vi "PH_PPPA_PowerUnit.ProcCases.vi"(0 "i ref in":refnum<vi>, 1 "selector":string, 2 "Data":T1, 3 "call cluster":T2={"Object"="", "Selector"="", "CallType"=enum."synchronous", "Async Object"="", "Async Selector"="", "Data Descriptor"="", "Data"=[], "Error #"=0, "Expire"=0}, 5 "error in (no error)":errorcluster) -> (14 "i ref out":refnum<vi>, 17 "answer cluster":T2={"Object"="", "Selector"="", "CallType"=enum."synchronous", "Async Object"="", "Async Selector"="", "Data Descriptor"="", "Data"=[], "Error #"=0, "Expire"=0}, 19 "error out":errorcluster)   [LabVIEW 2014, in "PH_PPPA_PowerUnit.lvlib"]
doc: "This method is called by a process from within the default case in the event loop. The methods of a class that are linked to events will be called from THIS method. Add your code here."
uses:
  PH_PPPA_PowerUnit.lvlib
  CSCore/CSSystem/CoreDefs/CoreDefs.call_type.ctl
  CSCore/BaseProcess/BaseProcess.descriptor string definition.ctl
  CSCore/CSSystem/CoreDefs/CoreDefs.rawDataType.ctl
  PH_PowerUnit_BaseClass/PH_PowerUnit_BaseClass.SM States.ctl
  CSCore/CSSystem/CoreLib/CoreLib.string 2 byte array.vi
  CSCore/CSSystem/CoreLib/CoreLib.byte array 2 double.vi
  CSCore/CSSystem/CoreLib/CoreLib.byte array 2 short.vi
  CSCore/BaseProcess/BaseProcess.lvlib
  CSCore/CSSystem/CoreLib/CoreLib.lvlib
  CSCore/CAEObj/CAEObj.lvlib
  PH_Common/PH_Common.lvlib
  PH_StatusHandler/PH_StatusHandler.lvlib
  PH_PSDBWriter/PH_PSDBWriter.lvlib
  CSCore/BaseSM/BaseSM.lvlib
  PH_PowerUnit_BaseClass/PH_PowerUnit_BaseClass.lvlib
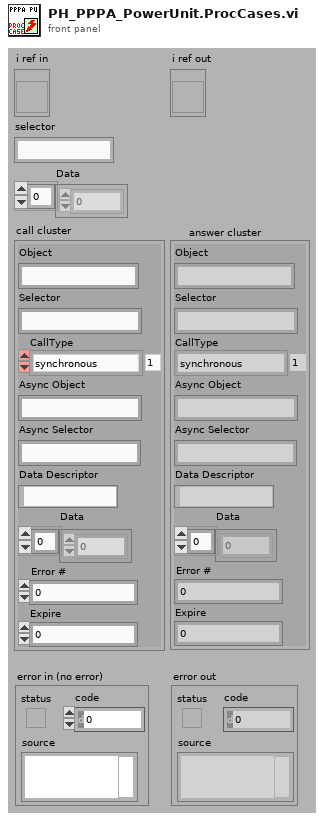
[diagram p1: front panel]
types:
  T1 = typedef "CoreDefs.rawDataType.ctl" = i8[]
  T2 = typedef "CoreDefs.call_type.ctl" = cluster{"Object":string, "Selector":string, "CallType":enum16{"simple", "synchronous", "asynchronous"}, "Async Object":string, "Async Selector":string, "Data Descriptor":T3, "Data":T1, "Error #":i32, "Expire":u32}
  T3 = typedef "BaseProcess.lvlib/BaseProcess.descriptor string definition.ctl" = string
  T4 = typedef "PH_PowerUnit_BaseClass.lvlib/PH_PowerUnit_BaseClass.SM States.ctl" = enum16{".", "Stand by", "Switch PU on", "Configure", "Set Default Voltage", "Set STANDBY", "Set READY", "Wait for Shot Cmd", "Open Dump Rods", "Open Ross Relais", "Close Ross Relais", "Switch PSU on", "Switch PSU off", "Charge", "Switch GD Channel on", "Close Dump Rods", "Rods-TO", "RR-TO", "PSU-TO", "Trigger-TO"}
  T5 = typedef "PH_PowerUnit_BaseClass.lvlib/PH_PowerUnit_BaseClass.i attribute.ctl" = cluster{"Constructor finished":bool, "PU":cluster{"In use":bool, "Service ID in use":i32, "GUI Ref":refnum<vi>}, "Enabling":cluster{"State":T6, "GUI Ref":refnum<vi>}, "Timing":cluster{"Last Shot":dbl, "Time between Shots [Sec]":dbl, "Waiting Time over?":bool, "Service ID Waiting Time":i32, "GUI Ref":refnum<vi>, "Instance":cluster{"Status":T7, "linked?":bool, "GUI Ref":refnum<vi>}}, "Sequencer":cluster{"SM State":string, "GUI Ref":refnum<vi>, "linked":bool}, "Subscribed Trendmssgs":cluster{"Tagname":string, "Status":T7, "linked?":bool, "Shot Condition":T7, "GUI Ref":refnum<vi>}[], "PP PU":T8, "Default Voltage (V)":dbl, "GUI Refs":T9, "PSDB data":cluster{"Shot Voltage [V]":dbl, "State TO SM":T4, "Write 2 early":bool}, "State TO SM":T4}
  T6 = typedef "PH_SystemInformation.lvlib/PH_SystemInformationEnabling State.ctl" = i32
  T7 = typedef "PH_StatusHandler.lvlib/PH_StatusHandler.Status.ctl" = i16
  T8 = typedef "PH_PP_Common.lvlib/PH_PP_Common.PUs.ctl" = enum16{"no Info", "PA-19mm-1", "PA-19mm-2", "PA-45mm-PILC", "PA-45mm-MAIN", "MA-PU-1", "MA-PU-2", "MA-PU-3", "MA-PU-4", "MA-PU-5", "MA-PU-6", "MA-FR", "MA-PILC", "PA-45mm-DP"}
  T9 = typedef "PH_PowerUnit_BaseClass.lvlib/PH_PowerUnit_BaseClass.GUI Refs.ctl" = cluster{"Delete Inst":refnum<vi>, "State TO SM":refnum<vi>, "State SM":refnum<vi>, "Fire":refnum<vi>}
  T10 = typedef "PH_PPPA_PowerUnit.lvlib/PH_PPPA_PowerUnit.i attribute.ctl" = cluster{"GUI Refs":cluster{"Ignitron":refnum<vi>, "Rossrelais":refnum<vi>, "Set Voltage":refnum<vi>, "PSU":refnum<vi>, "EOC":refnum<vi>, "Trigger":refnum<vi>}, "Ignitron":T11, "PSU":T12, "Dump Ross Relais":T13, "Trigger":cluster{"State Device":T7, "linked?":bool}, "Timing Settings":cluster{"Prdc Fast?":bool, "Default Value Periodic Interval":i32, "Mercury on since":dbl, "Warm up Time Mercury [s]":dbl}, "Set Voltage [V]":dbl, "19er Ignitionbox":string}
  T11 = typedef "PH_PP_Common.lvlib/PH_PP_Common.Ignitron Attributes.ctl" = cluster{"State Device":T7, "linked?":bool}
  T12 = typedef "PH_PP_Common.lvlib/PH_PP_Common.PSU Attributes.ctl" = cluster{"lower limit [V]":dbl, "upper limit [V]":dbl, "Voltage set":bool, "State Device":T7, "linked?":bool}
  T13 = typedef "PH_PP_Common.lvlib/PH_PP_Common.Ross Relais Attributes.ctl" = cluster{"State Device":T7, "linked?":bool}
  T14 = typedef "PH_PSDBWriter.lvlib/PH_PSDBWriter.PHELIX-Subsystems.ctl" = i32
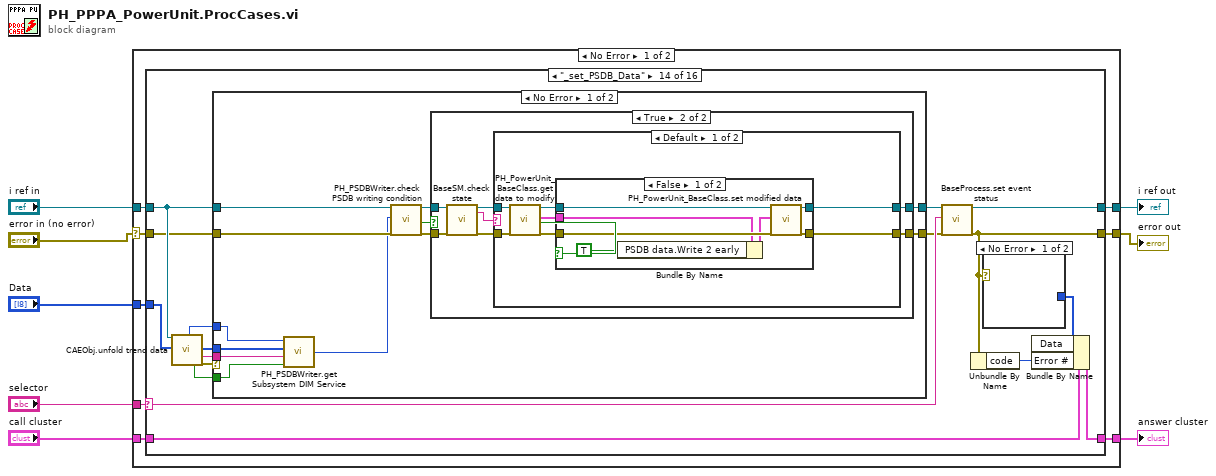
[diagram p0: block diagram]
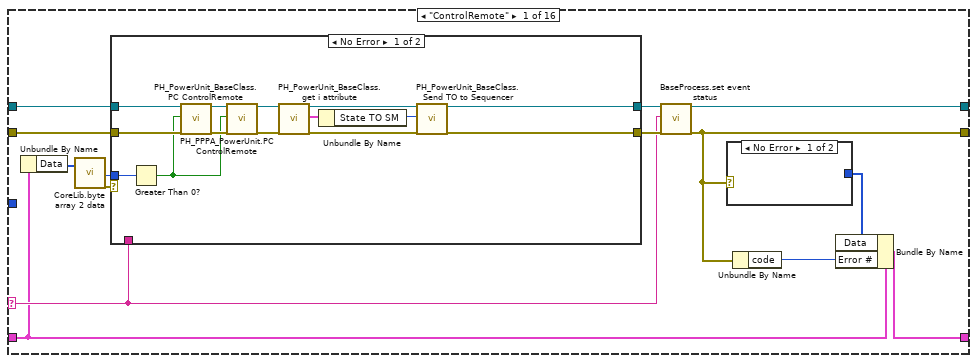
[diagram p2: hidden frame]
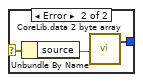
[diagram p3: hidden frame]
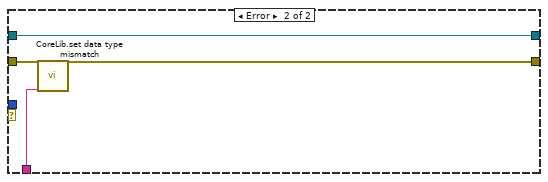
[diagram p4: hidden frame]
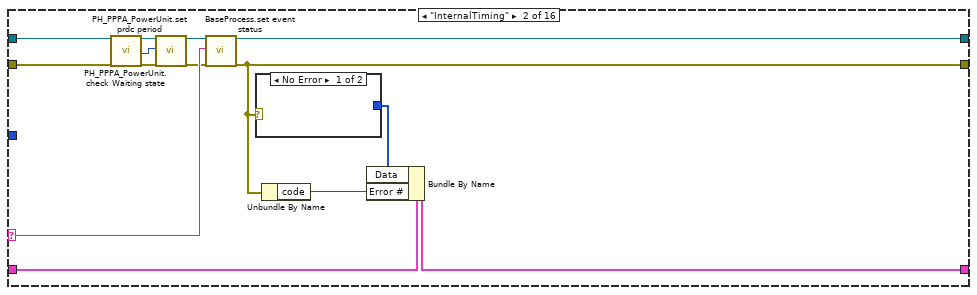
[diagram p5: hidden frame]
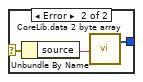
[diagram p6: hidden frame]
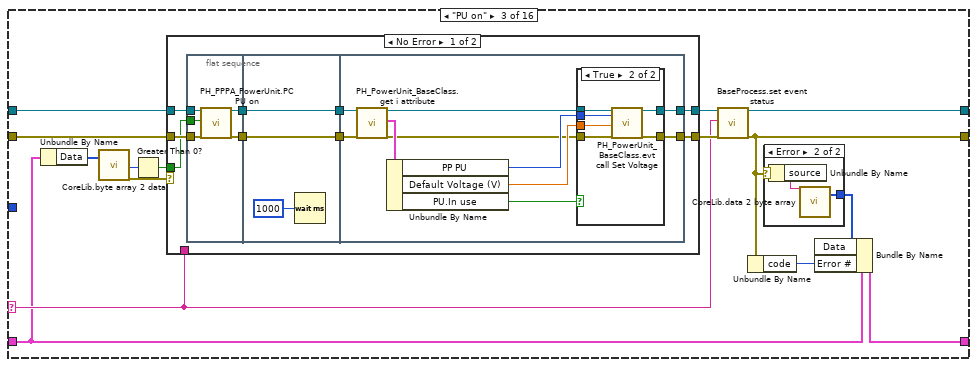
[diagram p7: hidden frame]
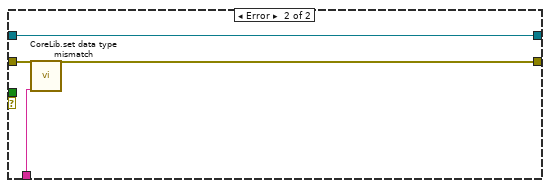
[diagram p10: hidden frame]
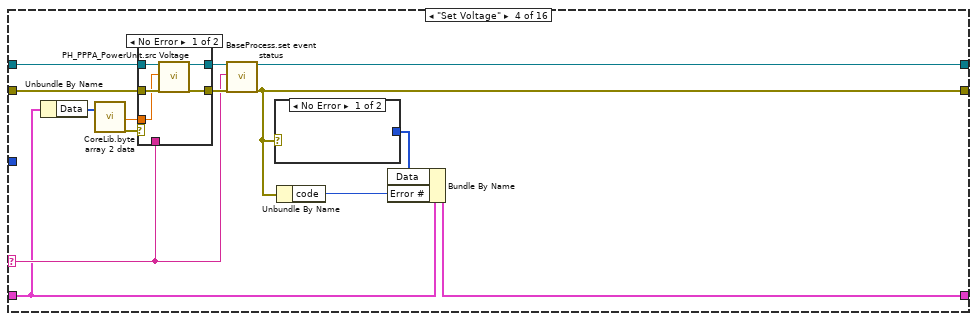
[diagram p11: hidden frame]
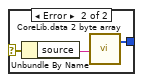
[diagram p12: hidden frame]
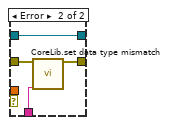
[diagram p13: hidden frame]
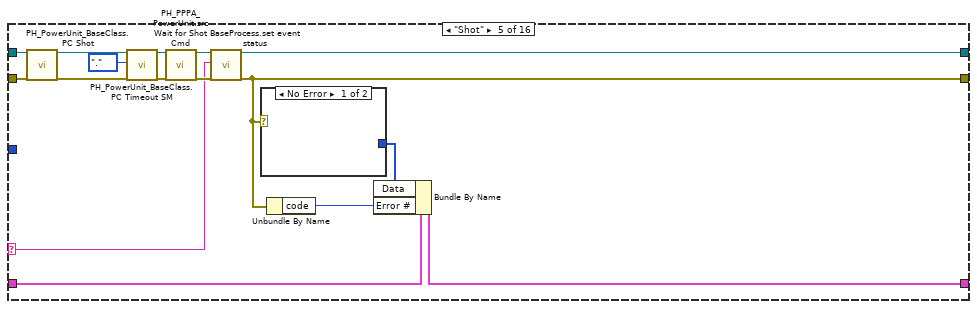
[diagram p14: hidden frame]
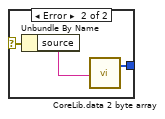
[diagram p15: hidden frame]
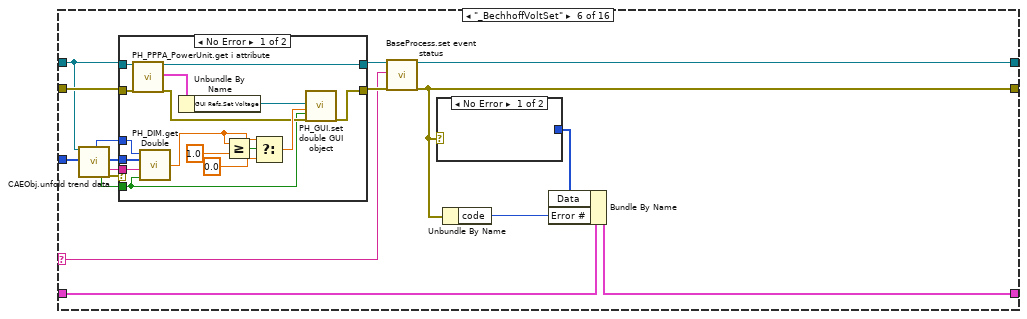
[diagram p16: hidden frame]
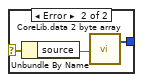
[diagram p17: hidden frame]
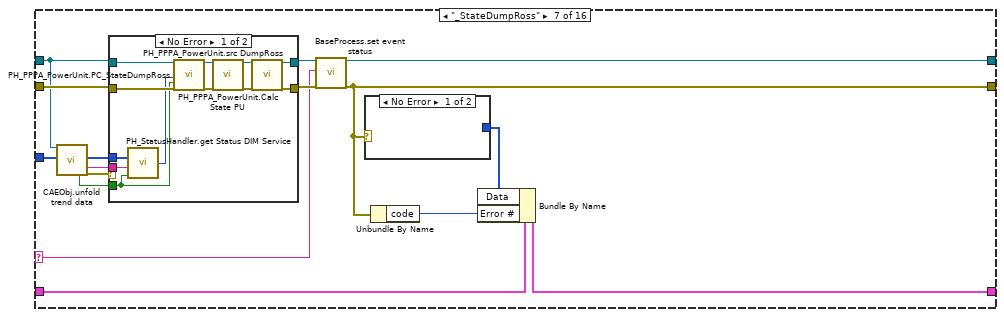
[diagram p19: hidden frame]
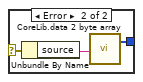
[diagram p20: hidden frame]
diagram:
  n1 = case shown="No Error" "error in (no error)" {
    selector: "error in (no error)" -> [w9 w589]
    tunnel: "selector" -> [w16 _]
    tunnel: [w15 w588] -> w7
    tunnel: "call cluster" -> [w14 w588]
    tunnel: "i ref in" -> [w13 w590]
    tunnel: [w12 w590] -> w4
    tunnel: [w11 w589] -> w3
    tunnel: "Data" -> [w10 _]
    frame No Error {
      n2 = case shown="\"_set_PSDB_Data\"" w16 {
        selector: w16 -> [w19 w60 w75 w133 w155 w180 w217 w250 w285 w338 w375 w404 w436 w489 w555 w580]
        tunnel: w13 -> [w30 w57 w83 w139 w167 w176 w213 w246 w279 w334 w369 w402 w435 w482 w548 w585]
        tunnel: [w21 w62 w77 w132 w157 w182 w220 w252 w287 w340 w374 w408 w440 w493 w559 w584] -> w12
        tunnel: w14 -> [w18 w59 w74 w130 w154 w179 w216 w249 w284 w337 w372 w406 w438 w491 w557 w578]
        tunnel: [w17 w58 w73 w129 w153 w178 w215 w248 w283 w336 w371 w405 w437 w490 w556 w581] -> w15
        tunnel: w9 -> [w29 w56 w82 w138 w166 w187 w224 w257 w278 w333 w380 w413 w445 w481 w547 w583]
        tunnel: [w20 w61 w76 w131 w156 w181 w219 w251 w286 w339 w373 w407 w439 w492 w558 w582] -> w11
        tunnel: w10 -> [_ _ _ _ _ w177 w214 w247 w282 w335 w370 w403 w434 w483 w549 w579]
        frame "ControlRemote" {
          n3 = Unbundle By Name(w18) -> ("Data"=w28:T1)
          n4 = call-poly "CoreLib.byte array 2 data.vi"("byteArray"=w28) -> ("i16"=w26:i16, "error out"=w27:errorcluster)  [unwired: 16 in, 1 out]
          n5 = case shown="No Error" w27 {
            tunnel: [w42 w51] -> w22
            tunnel: w30 -> [w47 w51]
            tunnel: w29 -> [w46 w50]
            tunnel: [w41 w49] -> w23
            tunnel: w19 -> [_ w48]
            tunnel: w26 -> [w35 _]
            frame No Error {
              n6 = Greater Than 0?(x=w35) -> (x > 0?=w34:bool)
              n7 = call "PH_PPPA_PowerUnit.PC ControlRemote.vi"("i ref in"=w47, "Remote Controlled?"=w34, "error in (no error)"=w46) -> ("i ref out"=w39:refnum<vi>, "error out"=w37:errorcluster)  [unwired: 15 in]
              n8 = call "PH_PowerUnit_BaseClass.PC ControlRemote.vi"("i ref in"=w39, "Remote controlled?"=w34, "error in (no error)"=w37) -> ("i ref out"=w38:refnum<vi>, "error out"=w36:errorcluster)  [unwired: 15 in]
              n9 = call "PH_PowerUnit_BaseClass.get i attribute.vi"("i ref in"=w38, "error in (no error)"=w36) -> ("i ref out"=w44:refnum<vi>, "i attribute"=w45:T5, "error out"=w40:errorcluster)  [unwired: 15 in]
              n10 = Unbundle By Name(w45) -> ("State TO SM"=w43:T4)
              n11 = call "PH_PowerUnit_BaseClass.Send TO to Sequencer.vi"("VI in"=w44, "State TO SM"=w43, "error in (no error)"=w40) -> ("VI out"=w42:refnum<vi>, "error out"=w41:errorcluster)  [unwired: 15 in]
            }
            frame Error {
              n12 = call "CoreLib.set data type mismatch.vi"("error in (no error)"=w50, "error source"=w48) -> ("error out"=w49:errorcluster)  [unwired: 17 in]
            }
          }
          n13 = call "BaseProcess.set event status.vi"("i ref in"=w22, "EventStatus"=w19, "error in (no error)"=w23) -> ("i ref out"=w21:refnum<vi>, "error out"=w20:errorcluster)  [unwired: 14 in, 1 out]
          n14 = case shown="No Error" w20 {
            selector: w20 -> [_ w33]
            tunnel: [_ w31] -> w24
            frame No Error {
            }
            frame Error {
              n15 = Unbundle By Name(w33) -> ("source"=w32:string)
              n16 = call-poly "CoreLib.data 2 byte array.vi"("string"=w32) -> ("byteArray out"=w31:T1)  [unwired: 18 in]
            }
          }
          n17 = Unbundle By Name(w20) -> ("code"=w25:i32)
          n18 = Bundle By Name(cluster=w18, "Data"=w24, "Error #"=w25) -> (w17:T2)
        }
        frame "InternalTiming" {
          n19 = call "PH_PPPA_PowerUnit.check Waiting state.vi"("i ref in"=w57, "error in (no error)"=w56) -> ("i ref out"=w55:refnum<vi>, "Waiting Time (s)"=w65:i32, "error out"=w54:errorcluster)  [unwired: 15 in]
          n20 = call "PH_PPPA_PowerUnit.set  prdc period.vi"("i ref in"=w55, "Waiting Time (s)"=w65, "error in (no error)"=w54) -> ("i ref out"=w53:refnum<vi>, "error out"=w52:errorcluster)  [unwired: 15 in]
          n21 = call "BaseProcess.set event status.vi"("i ref in"=w53, "EventStatus"=w60, "error in (no error)"=w52) -> ("i ref out"=w62:refnum<vi>, "error out"=w61:errorcluster)  [unwired: 14 in, 1 out]
          n22 = case shown="No Error" w61 {
            selector: w61 -> [_ w68]
            tunnel: [_ w66] -> w63
            frame No Error {
            }
            frame Error {
              n23 = Unbundle By Name(w68) -> ("source"=w67:string)
              n24 = call-poly "CoreLib.data 2 byte array.vi"("string"=w67) -> ("byteArray out"=w66:T1)  [unwired: 18 in]
            }
          }
          n25 = Unbundle By Name(w61) -> ("code"=w64:i32)
          n26 = Bundle By Name(cluster=w59, "Data"=w63, "Error #"=w64) -> (w58:T2)
        }
        frame "PU on" {
          n27 = Unbundle By Name(w74) -> ("Data"=w72:T1)
          n28 = call-poly "CoreLib.byte array 2 data.vi"("byteArray"=w72) -> ("i16"=w71:i16, "error out"=w69:errorcluster)  [unwired: 16 in, 1 out]
          n29 = Greater Than 0?(x=w71) -> (x > 0?=w70:bool)
          n30 = case shown="No Error" w69 {
            tunnel: w83 -> [w95 w123]
            tunnel: [w93 w123] -> w78
            tunnel: w82 -> [w94 w125]
            tunnel: [w92 w124] -> w79
            tunnel: w75 -> [_ w122]
            tunnel: w70 -> [w91 _]
            frame No Error {
              n31 = flat-sequence {
                tunnel: w95 -> [w100]
                tunnel: w94 -> [w99]
                tunnel: w91 -> [w96]
                tunnel: [w98] -> w90
                tunnel: [w97] -> w89
                tunnel: w90 -> [w103]
                tunnel: w89 -> [w102]
                tunnel: [w103] -> w88
                tunnel: [w102] -> w87
                tunnel: [w110] -> w92
                tunnel: [w111] -> w93
                tunnel: w88 -> [w113]
                tunnel: w87 -> [w112]
                frame #0 {
                  n32 = call "PH_PPPA_PowerUnit.PC PU on.vi"("i ref in"=w100, "PU on"=w96, "error in (no error)"=w99) -> ("i ref out"=w98:refnum<vi>, "error out"=w97:errorcluster)  [unwired: 15 in]
                }
                frame #1 {
                  n33 = Wait (ms)(milliseconds to wait=u32 1000) -> ()  [unwired: 1 out]
                }
                frame #2 {
                  n34 = call "PH_PowerUnit_BaseClass.get i attribute.vi"("i ref in"=w113, "error in (no error)"=w112) -> ("i ref out"=w105:refnum<vi>, "i attribute"=w109:T5, "error out"=w104:errorcluster)  [unwired: 15 in]
                  n35 = Unbundle By Name(w109) -> ("PP PU"=w106:T8, "Default Voltage (V)"=w107:dbl, "PU.In use"=w108:bool)
                  n36 = case shown="True" w108 {
                    tunnel: w105 -> [w115 w121]
                    tunnel: [w115 w120] -> w111
                    tunnel: w104 -> [w114 w119]
                    tunnel: [w114 w118] -> w110
                    tunnel: w107 -> [_ w117]
                    tunnel: w106 -> [_ w116]
                    frame False {
                    }
                    frame True {
                      n37 = call "PH_PowerUnit_BaseClass.evt call Set Voltage.vi"("i ref in"=w121, "PowerUnit"=w116, "Voltage [V]"=w117, "error in (no error)"=w119) -> ("i ref out"=w120:refnum<vi>, "error out"=w118:errorcluster)  [unwired: 14 in]
                    }
                  }
                }
              }
            }
            frame Error {
              n38 = call "CoreLib.set data type mismatch.vi"("error in (no error)"=w125, "error source"=w122) -> ("error out"=w124:errorcluster)  [unwired: 17 in]
            }
          }
          n39 = call "BaseProcess.set event status.vi"("i ref in"=w78, "EventStatus"=w75, "error in (no error)"=w79) -> ("i ref out"=w77:refnum<vi>, "error out"=w76:errorcluster)  [unwired: 14 in, 1 out]
          n40 = Unbundle By Name(w76) -> ("code"=w81:i32)
          n41 = case shown="Error" w76 {
            selector: w76 -> [_ w86]
            tunnel: [_ w84] -> w80
            frame No Error {
            }
            frame Error {
              n42 = Unbundle By Name(w86) -> ("source"=w85:string)
              n43 = call-poly "CoreLib.data 2 byte array.vi"("string"=w85) -> ("byteArray out"=w84:T1)  [unwired: 18 in]
            }
          }
          n44 = Bundle By Name(cluster=w74, "Data"=w80, "Error #"=w81) -> (w73:T2)
        }
        frame "Set Voltage" {
          n45 = Unbundle By Name(w130) -> ("Data"=w128:T1)
          n46 = call-poly "CoreLib.byte array 2 data.vi"("byteArray"=w128) -> ("d64"=w127:dbl, "error out"=w126:errorcluster)  [unwired: 16 in, 1 out]
          n47 = case shown="No Error" w126 {
            tunnel: w139 -> [w147 w149]
            tunnel: [w145 w149] -> w134
            tunnel: w138 -> [w146 w151]
            tunnel: [w144 w150] -> w135
            tunnel: w133 -> [_ w148]
            tunnel: w127 -> [w143 _]
            frame No Error {
              n48 = call "PH_PPPA_PowerUnit.src Voltage.vi"("i ref in"=w147, "Voltage [V]"=w143, "error in (no error)"=w146) -> ("i ref out"=w145:refnum<vi>, "error out"=w144:errorcluster)  [unwired: 15 in]
            }
            frame Error {
              n49 = call "CoreLib.set data type mismatch.vi"("error in (no error)"=w151, "error source"=w148) -> ("error out"=w150:errorcluster)  [unwired: 17 in]
            }
          }
          n50 = call "BaseProcess.set event status.vi"("i ref in"=w134, "EventStatus"=w133, "error in (no error)"=w135) -> ("i ref out"=w132:refnum<vi>, "error out"=w131:errorcluster)  [unwired: 14 in, 1 out]
          n51 = case shown="No Error" w131 {
            selector: w131 -> [_ w142]
            tunnel: [_ w140] -> w136
            frame No Error {
            }
            frame Error {
              n52 = Unbundle By Name(w142) -> ("source"=w141:string)
              n53 = call-poly "CoreLib.data 2 byte array.vi"("string"=w141) -> ("byteArray out"=w140:T1)  [unwired: 18 in]
            }
          }
          n54 = Unbundle By Name(w131) -> ("code"=w137:i32)
          n55 = Bundle By Name(cluster=w130, "Data"=w136, "Error #"=w137) -> (w129:T2)
        }
        frame "Shot" {
          n56 = call "PH_PowerUnit_BaseClass.PC Shot.vi"("i ref in"=w167, "error in (no error)"=w166) -> ("i ref out"=w165:refnum<vi>, "error out"=w164:errorcluster)  [unwired: 16 in]
          n57 = call "PH_PowerUnit_BaseClass.PC Timeout SM.vi"("VI in"=w165, "Timeout SM"=PH_PowerUnit_BaseClass.SM_States.".", "error in (no error)"=w164) -> ("VI out"=w162:refnum<vi>, "error out"=w163:errorcluster)  [unwired: 15 in]
          n58 = call "PH_PPPA_PowerUnit.src Wait for Shot Cmd.vi"("i ref in"=w162, "error in (no error)"=w163) -> ("i ref out"=w158:refnum<vi>, "error out"=w159:errorcluster)  [unwired: 16 in]
          n59 = call "BaseProcess.set event status.vi"("i ref in"=w158, "EventStatus"=w155, "error in (no error)"=w159) -> ("i ref out"=w157:refnum<vi>, "error out"=w156:errorcluster)  [unwired: 14 in, 1 out]
          n60 = case shown="No Error" w156 {
            selector: w156 -> [_ w170]
            tunnel: [_ w168] -> w160
            frame No Error {
            }
            frame Error {
              n61 = Unbundle By Name(w170) -> ("source"=w169:string)
              n62 = call-poly "CoreLib.data 2 byte array.vi"("string"=w169) -> ("byteArray out"=w168:T1)  [unwired: 18 in]
            }
          }
          n63 = Unbundle By Name(w156) -> ("code"=w161:i32)
          n64 = Bundle By Name(cluster=w154, "Data"=w160, "Error #"=w161) -> (w153:T2)
        }
        frame "_BechhoffVoltSet" {
          n65 = call "CAEObj.unfold trend data.vi"("i ref in"=w176, "raw trend data"=w177) -> ("quality"=w171:i32, "no link"=w172:bool, "data"=w173:i8[], "typeDescriptor"=w174:string, "error out"=w175:errorcluster)  [unwired: 9 in, 4 out]
          n66 = case shown="No Error" w175 {
            tunnel: w176 -> [w206 w208]
            tunnel: [w201 w208] -> w183
            tunnel: w187 -> [w205 w207]
            tunnel: [w192 w207] -> w184
            tunnel: w174 -> [w198 _]
            tunnel: w173 -> [w197 _]
            tunnel: w172 -> [w191 _]
            tunnel: w171 -> [w196 _]
            frame No Error {
              n67 = call "PH_PPPA_PowerUnit.get i attribute.vi"("i ref in"=w206, "error in (no error)"=w205) -> ("i ref out"=w201:refnum<vi>, "i attribute"=w204:T10, "error out"=w193:errorcluster)  [unwired: 15 in]
              n68 = call "PH_DIM.get Double.vi"("no link"=w191, "typeDescriptor"=w198, "data"=w197, "quality"=w196) -> ("Value"=w200:dbl)
              n69 = Unbundle By Name(w204) -> ("GUI Refs.Set Voltage"=w194:refnum<vi>)
              n70 = Greater Or Equal?(x=w200, y=1.0) -> (x >= y?=w199:bool)
              n71 = Select(t=w200, s=w199, f=0.0) -> (s? t:f=w195:dbl)
              n72 = call "PH_GUI.set double GUI object.vi"("GUI object Ref"=w194, "value"=w195, "blinking (false)"=w191, "error in (no error)"=w193) -> ("error out"=w192:errorcluster)  [unwired: 15 in]
            }
            frame Error {
            }
          }
          n73 = call "BaseProcess.set event status.vi"("i ref in"=w183, "EventStatus"=w180, "error in (no error)"=w184) -> ("i ref out"=w182:refnum<vi>, "error out"=w181:errorcluster)  [unwired: 14 in, 1 out]
          n74 = case shown="No Error" w181 {
            selector: w181 -> [_ w190]
            tunnel: [_ w188] -> w185
            frame No Error {
            }
            frame Error {
              n75 = Unbundle By Name(w190) -> ("source"=w189:string)
              n76 = call-poly "CoreLib.data 2 byte array.vi"("string"=w189) -> ("byteArray out"=w188:T1)  [unwired: 18 in]
            }
          }
          n77 = Unbundle By Name(w181) -> ("code"=w186:i32)
          n78 = Bundle By Name(cluster=w179, "Data"=w185, "Error #"=w186) -> (w178:T2)
        }
        frame "_StateDumpRoss" {
          n79 = call "CAEObj.unfold trend data.vi"("i ref in"=w213, "raw trend data"=w214) -> ("no link"=w209:bool, "data"=w211:i8[], "typeDescriptor"=w212:string, "error out"=w210:errorcluster)  [unwired: 9 in, 5 out]
          n80 = case shown="No Error" w210 {
            tunnel: w213 -> [w239 w241]
            tunnel: [w233 w241] -> w218
            tunnel: w224 -> [w238 w240]
            tunnel: [w234 w240] -> w221
            tunnel: w212 -> [w237 _]
            tunnel: w211 -> [w236 _]
            tunnel: w209 -> [w228 _]
            frame No Error {
              n81 = call "PH_StatusHandler.get Status DIM Service.vi"("no link"=w228, "typeDescriptor"=w237, "data"=w236) -> ("Status"=w235:T7)  [unwired: 1 in]
              n82 = call "PH_PPPA_PowerUnit.PC_StateDumpRoss.vi"("i ref in"=w239, "Dump Ross State"=w235, "not linked"=w228, "error in (no error)"=w238) -> ("i ref out"=w232:refnum<vi>, "error out"=w230:errorcluster)  [unwired: 14 in]
              n83 = call "PH_PPPA_PowerUnit.Calc State PU.vi"("i ref in"=w232, "error in (no error)"=w230) -> ("i ref out"=w231:refnum<vi>, "error out"=w229:errorcluster)  [unwired: 16 in]
              n84 = call "PH_PPPA_PowerUnit.src DumpRoss.vi"("i ref in"=w231, "error in (no error)"=w229) -> ("i ref out"=w233:refnum<vi>, "error out"=w234:errorcluster)  [unwired: 16 in]
            }
            frame Error {
            }
          }
          n85 = call "BaseProcess.set event status.vi"("i ref in"=w218, "EventStatus"=w217, "error in (no error)"=w221) -> ("i ref out"=w220:refnum<vi>, "error out"=w219:errorcluster)  [unwired: 14 in, 1 out]
          n86 = case shown="No Error" w219 {
            selector: w219 -> [_ w227]
            tunnel: [_ w225] -> w222
            frame No Error {
            }
            frame Error {
              n87 = Unbundle By Name(w227) -> ("source"=w226:string)
              n88 = call-poly "CoreLib.data 2 byte array.vi"("string"=w226) -> ("byteArray out"=w225:T1)  [unwired: 18 in]
            }
          }
          n89 = Unbundle By Name(w219) -> ("code"=w223:i32)
          n90 = Bundle By Name(cluster=w216, "Data"=w222, "Error #"=w223) -> (w215:T2)
        }
        frame "_StateIgni" {
          n91 = call "CAEObj.unfold trend data.vi"("i ref in"=w246, "raw trend data"=w247) -> ("no link"=w242:bool, "data"=w244:i8[], "typeDescriptor"=w243:string, "error out"=w245:errorcluster)  [unwired: 9 in, 5 out]
          n92 = case shown="No Error" w245 {
            tunnel: w246 -> [w268 w272]
            tunnel: [w270 w272] -> w253
            tunnel: w257 -> [w266 w271]
            tunnel: [w269 w271] -> w254
            tunnel: w244 -> [w264 _]
            tunnel: w243 -> [w263 _]
            tunnel: w242 -> [w261 _]
            frame No Error {
              n93 = call "PH_StatusHandler.get Status DIM Service.vi"("no link"=w261, "typeDescriptor"=w263, "data"=w264) -> ("Status"=w262:T7)  [unwired: 1 in]
              n94 = call "PH_PPPA_PowerUnit.PC_StateIgni.vi"("i ref in"=w268, "Igni Status"=w262, "not linked?"=w261, "error in (no error)"=w266) -> ("i ref out"=w267:refnum<vi>, "error out"=w265:errorcluster)  [unwired: 14 in]
              n95 = call "PH_PPPA_PowerUnit.Calc State PU.vi"("i ref in"=w267, "error in (no error)"=w265) -> ("i ref out"=w270:refnum<vi>, "error out"=w269:errorcluster)  [unwired: 16 in]
            }
            frame Error {
            }
          }
          n96 = call "BaseProcess.set event status.vi"("i ref in"=w253, "EventStatus"=w250, "error in (no error)"=w254) -> ("i ref out"=w252:refnum<vi>, "error out"=w251:errorcluster)  [unwired: 14 in, 1 out]
          n97 = case shown="No Error" w251 {
            selector: w251 -> [_ w260]
            tunnel: [_ w258] -> w255
            frame No Error {
            }
            frame Error {
              n98 = Unbundle By Name(w260) -> ("source"=w259:string)
              n99 = call-poly "CoreLib.data 2 byte array.vi"("string"=w259) -> ("byteArray out"=w258:T1)  [unwired: 18 in]
            }
          }
          n100 = Unbundle By Name(w251) -> ("code"=w256:i32)
          n101 = Bundle By Name(cluster=w249, "Data"=w255, "Error #"=w256) -> (w248:T2)
        }
        frame "_MercuryOnSince" {
          n102 = call "CAEObj.unfold trend data.vi"("i ref in"=w279, "raw trend data"=w282) -> ("quality"=w277:i32, "no link"=w276:bool, "data"=w273:i8[], "typeDescriptor"=w274:string, "error out"=w275:errorcluster)  [unwired: 9 in, 4 out]
          n103 = case shown="No Error" w275 {
            tunnel: w279 -> [w302 w322]
            tunnel: [w297 w322] -> w280
            tunnel: w278 -> [w301 w321]
            tunnel: [w295 w321] -> w281
            tunnel: w273 -> [w300 _]
            tunnel: w274 -> [w299 _]
            tunnel: w276 -> [w290 _]
            tunnel: w277 -> [w294 _]
            frame No Error {
              n104 = call "PH_PPPA_PowerUnit.get data to modify.vi"("i ref in"=w302, "error in (no error)"=w301) -> ("i ref out"=w298:refnum<vi>, "i attribute"=w291:T10, "timed out"=w292:bool, "error out"=w296:errorcluster)  [unwired: 14 in]
              n105 = call "PH_DIM.get String.vi"("no link"=w290, "typeDescriptor"=w299, "data"=w300, "quality"=w294) -> ("Output String"=w293:string)
              n106 = case shown="False" w292 {
                tunnel: w298 -> [w311 w320]
                tunnel: [w310 w320] -> w297
                tunnel: w296 -> [w309 w319]
                tunnel: [w308 w319] -> w295
                tunnel: w293 -> [w307 _]
                tunnel: w291 -> [w306 _]
                tunnel: w290 -> [w304 _]
                frame False {
                  n107 = case shown="False" w304 {
                    tunnel: w307 -> [w314 _]
                    tunnel: [w313 9999.0] -> w303
                    frame False {
                      n108 = Match Pattern(string=w314, regular expression=" ") -> (before substring=w316:string, after substring=w315:string)  [unwired: 1 in, 2 out]
                      n109 = call "PH_Strings.convert Time 1.vi"("Date"=w316, "Time"=w315) -> ("Time"=w312:timestamp)
                      n110 = To Double Precision Float(number=w312) -> (double precision float=w313:dbl)
                    }
                    frame True {
                    }
                  }
                  n111 = Bundle By Name(cluster=w306, "Timing Settings.Mercury on since"=w303) -> (w305:T10)
                  n112 = call "PH_PPPA_PowerUnit.set modified data.vi"("i ref in"=w311, "i attribute"=w305, "error in (no error)"=w309) -> ("i ref out"=w310:refnum<vi>, "error out"=w308:errorcluster)  [unwired: 15 in]
                }
                frame True {
                }
              }
            }
            frame Error {
            }
          }
          n113 = call "BaseProcess.set event status.vi"("i ref in"=w280, "EventStatus"=w285, "error in (no error)"=w281) -> ("i ref out"=w287:refnum<vi>, "error out"=w286:errorcluster)  [unwired: 14 in, 1 out]
          n114 = case shown="No Error" w286 {
            selector: w286 -> [_ w325]
            tunnel: [_ w323] -> w288
            frame No Error {
            }
            frame Error {
              n115 = Unbundle By Name(w325) -> ("source"=w324:string)
              n116 = call-poly "CoreLib.data 2 byte array.vi"("string"=w324) -> ("byteArray out"=w323:T1)  [unwired: 18 in]
            }
          }
          n117 = Unbundle By Name(w286) -> ("code"=w289:i32)
          n118 = Bundle By Name(cluster=w284, "Data"=w288, "Error #"=w289) -> (w283:T2)
        }
        frame "_LastShot" {
          n119 = call "CAEObj.unfold trend data.vi"("i ref in"=w334, "raw trend data"=w335) -> ("quality"=w329:i32, "no link"=w330:bool, "data"=w328:i8[], "typeDescriptor"=w326:string, "error out"=w327:errorcluster)  [unwired: 9 in, 4 out]
          n120 = case shown="No Error" w327 {
            tunnel: w334 -> [w344 w361]
            tunnel: [w350 w361] -> w332
            tunnel: w333 -> [w343 w360]
            tunnel: [w349 w360] -> w331
            tunnel: w328 -> [w352 _]
            tunnel: w326 -> [w351 _]
            tunnel: w330 -> [w346 _]
            tunnel: w329 -> [w348 _]
            frame No Error {
              n121 = call "PH_DIM.get String.vi"("no link"=w346, "typeDescriptor"=w351, "data"=w352, "quality"=w348) -> ("Output String"=w347:string)
              n122 = case shown="False" w346 {
                tunnel: w347 -> [w355 _]
                tunnel: [w353 9999.0] -> w345
                frame False {
                  n123 = Match Pattern(string=w355, regular expression=" ") -> (before substring=w357:string, after substring=w356:string)  [unwired: 1 in, 2 out]
                  n124 = call "PH_Strings.convert Time 1.vi"("Date"=w357, "Time"=w356) -> ("Time"=w354:timestamp)
                  n125 = To Double Precision Float(number=w354) -> (double precision float=w353:dbl)
                }
                frame True {
                }
              }
              n126 = call "PH_PowerUnit_BaseClass.set Last Shot.vi"("VI in"=w344, "Last Shot"=w345, "error in (no error)"=w343) -> ("VI out"=w350:refnum<vi>, "error out"=w349:errorcluster)  [unwired: 15 in]
            }
            frame Error {
            }
          }
          n127 = call "BaseProcess.set event status.vi"("i ref in"=w332, "EventStatus"=w338, "error in (no error)"=w331) -> ("i ref out"=w340:refnum<vi>, "error out"=w339:errorcluster)  [unwired: 14 in, 1 out]
          n128 = case shown="No Error" w339 {
            selector: w339 -> [_ w364]
            tunnel: [_ w362] -> w341
            frame No Error {
            }
            frame Error {
              n129 = Unbundle By Name(w364) -> ("source"=w363:string)
              n130 = call-poly "CoreLib.data 2 byte array.vi"("string"=w363) -> ("byteArray out"=w362:T1)  [unwired: 18 in]
            }
          }
          n131 = Unbundle By Name(w339) -> ("code"=w342:i32)
          n132 = Bundle By Name(cluster=w337, "Data"=w341, "Error #"=w342) -> (w336:T2)
        }
        frame "_StatePSU" {
          n133 = call "CAEObj.unfold trend data.vi"("i ref in"=w369, "raw trend data"=w370) -> ("no link"=w365:bool, "data"=w366:i8[], "typeDescriptor"=w367:string, "error out"=w368:errorcluster)  [unwired: 9 in, 5 out]
          n134 = case shown="No Error" w368 {
            tunnel: w369 -> [w395 w397]
            tunnel: [w388 w397] -> w376
            tunnel: w380 -> [w394 w396]
            tunnel: [w389 w396] -> w377
            tunnel: w367 -> [w393 _]
            tunnel: w366 -> [w392 _]
            tunnel: w365 -> [w390 _]
            frame No Error {
              n135 = call "PH_StatusHandler.get Status DIM Service.vi"("no link"=w390, "typeDescriptor"=w393, "data"=w392) -> ("Status"=w391:T7)  [unwired: 1 in]
              n136 = call "PH_PPPA_PowerUnit.PC_StatePSU.vi"("i ref in"=w395, "State PSU"=w391, "not linked?"=w390, "error in (no error)"=w394) -> ("i ref out"=w387:refnum<vi>, "error out"=w385:errorcluster)  [unwired: 14 in]
              n137 = call "PH_PPPA_PowerUnit.Calc State PU.vi"("i ref in"=w387, "error in (no error)"=w385) -> ("i ref out"=w386:refnum<vi>, "error out"=w384:errorcluster)  [unwired: 16 in]
              n138 = call "PH_PPPA_PowerUnit.src PSU.vi"("i ref in"=w386, "error in (no error)"=w384) -> ("i ref out"=w388:refnum<vi>, "error out"=w389:errorcluster)  [unwired: 16 in]
            }
            frame Error {
            }
          }
          n139 = call "BaseProcess.set event status.vi"("i ref in"=w376, "EventStatus"=w375, "error in (no error)"=w377) -> ("i ref out"=w374:refnum<vi>, "error out"=w373:errorcluster)  [unwired: 14 in, 1 out]
          n140 = case shown="No Error" w373 {
            selector: w373 -> [_ w383]
            tunnel: [_ w381] -> w378
            frame No Error {
            }
            frame Error {
              n141 = Unbundle By Name(w383) -> ("source"=w382:string)
              n142 = call-poly "CoreLib.data 2 byte array.vi"("string"=w382) -> ("byteArray out"=w381:T1)  [unwired: 18 in]
            }
          }
          n143 = Unbundle By Name(w373) -> ("code"=w379:i32)
          n144 = Bundle By Name(cluster=w372, "Data"=w378, "Error #"=w379) -> (w371:T2)
        }
        frame "_StateTrigger" {
          n145 = call "CAEObj.unfold trend data.vi"("i ref in"=w402, "raw trend data"=w403) -> ("no link"=w398:bool, "data"=w400:i8[], "typeDescriptor"=w399:string, "error out"=w401:errorcluster)  [unwired: 9 in, 5 out]
          n146 = case shown="No Error" w401 {
            tunnel: w402 -> [w428 w430]
            tunnel: [w421 w430] -> w409
            tunnel: w413 -> [w427 w429]
            tunnel: [w422 w429] -> w410
            tunnel: w400 -> [w426 _]
            tunnel: w399 -> [w425 _]
            tunnel: w398 -> [w423 _]
            frame No Error {
              n147 = call "PH_StatusHandler.get Status DIM Service.vi"("no link"=w423, "typeDescriptor"=w425, "data"=w426) -> ("Status"=w424:T7)  [unwired: 1 in]
              n148 = call "PH_PPPA_PowerUnit.PC_StateTrigger.vi"("i ref in"=w428, "Trigger Status"=w424, "not linked?"=w423, "error in (no error)"=w427) -> ("i ref out"=w420:refnum<vi>, "error out"=w418:errorcluster)  [unwired: 14 in]
              n149 = call "PH_PPPA_PowerUnit.Calc State PU.vi"("i ref in"=w420, "error in (no error)"=w418) -> ("i ref out"=w419:refnum<vi>, "error out"=w417:errorcluster)  [unwired: 16 in]
              n150 = call "PH_PPPA_PowerUnit.src Switch GD Channel on.vi"("i ref in"=w419, "error in (no error)"=w417) -> ("i ref out"=w421:refnum<vi>, "error out"=w422:errorcluster)  [unwired: 16 in]
            }
            frame Error {
            }
          }
          n151 = call "BaseProcess.set event status.vi"("i ref in"=w409, "EventStatus"=w404, "error in (no error)"=w410) -> ("i ref out"=w408:refnum<vi>, "error out"=w407:errorcluster)  [unwired: 14 in, 1 out]
          n152 = case shown="No Error" w407 {
            selector: w407 -> [_ w416]
            tunnel: [_ w414] -> w411
            frame No Error {
            }
            frame Error {
              n153 = Unbundle By Name(w416) -> ("source"=w415:string)
              n154 = call-poly "CoreLib.data 2 byte array.vi"("string"=w415) -> ("byteArray out"=w414:T1)  [unwired: 18 in]
            }
          }
          n155 = Unbundle By Name(w407) -> ("code"=w412:i32)
          n156 = Bundle By Name(cluster=w406, "Data"=w411, "Error #"=w412) -> (w405:T2)
        }
        frame "_setLimits" {
          n157 = call "CAEObj.unfold trend data.vi"("i ref in"=w435, "raw trend data"=w434) -> ("no link"=w431:bool, "data"=w433:i8[], "error out"=w432:errorcluster)  [unwired: 9 in, 6 out]
          n158 = case shown="No Error" w432 {
            tunnel: w435 -> [w450 w478]
            tunnel: [w456 w478] -> w441
            tunnel: w445 -> [w449 w477]
            tunnel: [w455 w477] -> w442
            tunnel: w433 -> [w452 _]
            tunnel: w431 -> [w451 _]
            frame No Error {
              n159 = case shown="False" w451 {
                tunnel: [w465 w466] -> w454
                tunnel: [w464 w466] -> w453
                tunnel: w452 -> [w462 _]
                frame False {
                  n160 = Type Cast(type=dbl[] [] ("array"), x=w462) -> (*(type *) &x=w463:dbl[])
                  n161 = Index Array(array=w463) -> (element #1=w465:dbl, element #2=w464:dbl)  [unwired: 2 in]
                }
                frame True {
                  w466 = 0.0 ("Numeric")
                }
              }
              n162 = call "PH_PPPA_PowerUnit.get data to modify.vi"("i ref in"=w450, "error in (no error)"=w449) -> ("i ref out"=w460:refnum<vi>, "i attribute"=w458:T10, "timed out"=w457:bool, "error out"=w459:errorcluster)  [unwired: 14 in]
              n163 = case shown="False" w457 {
                tunnel: w460 -> [w473 w476]
                tunnel: w459 -> [w472 w475]
                tunnel: w458 -> [w471 _]
                tunnel: w454 -> [w470 _]
                tunnel: w453 -> [w469 _]
                tunnel: [w468 w476] -> w456
                tunnel: [w467 w475] -> w455
                frame False {
                  n164 = Bundle By Name(cluster=w471, "PSU.lower limit [V]"=w470, "PSU.upper limit [V]"=w469) -> (w474:T10)
                  n165 = call "PH_PPPA_PowerUnit.set modified data.vi"("i ref in"=w473, "i attribute"=w474, "error in (no error)"=w472) -> ("i ref out"=w468:refnum<vi>, "error out"=w467:errorcluster)  [unwired: 15 in]
                }
                frame True {
                }
              }
            }
            frame Error {
            }
          }
          n166 = call "BaseProcess.set event status.vi"("i ref in"=w441, "EventStatus"=w436, "error in (no error)"=w442) -> ("i ref out"=w440:refnum<vi>, "error out"=w439:errorcluster)  [unwired: 14 in, 1 out]
          n167 = case shown="No Error" w439 {
            selector: w439 -> [_ w448]
            tunnel: [_ w446] -> w443
            frame No Error {
            }
            frame Error {
              n168 = Unbundle By Name(w448) -> ("source"=w447:string)
              n169 = call-poly "CoreLib.data 2 byte array.vi"("string"=w447) -> ("byteArray out"=w446:T1)  [unwired: 18 in]
            }
          }
          n170 = Unbundle By Name(w439) -> ("code"=w444:i32)
          n171 = Bundle By Name(cluster=w438, "Data"=w443, "Error #"=w444) -> (w437:T2)
        }
        frame "_set_PSDB_Data" {
          n172 = call "CAEObj.unfold trend data.vi"("i ref in"=w482, "raw trend data"=w483) -> ("quality"=w484:i32, "no link"=w487:bool, "data"=w485:i8[], "typeDescriptor"=w486:string, "error out"=w488:errorcluster)  [unwired: 9 in, 4 out]
          n173 = case shown="No Error" w488 {
            tunnel: w481 -> [w503 w541]
            tunnel: [w507 w540] -> w480
            tunnel: [w506 w541] -> w479
            tunnel: w482 -> [w505 w540]
            tunnel: w487 -> [w497 _]
            tunnel: w486 -> [w499 _]
            tunnel: w485 -> [w500 _]
            tunnel: w484 -> [w498 _]
            frame No Error {
              n174 = call "PH_PSDBWriter.get Subsystem DIM Service.vi"("no link"=w497, "typeDescriptor"=w499, "data"=w500, "quality"=w498) -> ("PHELIX Subsystems"=w496:T14)
              n175 = call "PH_PSDBWriter.check PSDB writing condition.vi"("i ref in"=w505, "wanted Subsystem"=w496, "error IO"=w503) -> ("i ref out"=w504:refnum<vi>, "write PSDB?"=w501:bool, "error out"=w502:errorcluster)  [unwired: 14 in]
              n176 = case shown="True" w501 {
                tunnel: w502 -> [w508 w512]
                tunnel: [w509 w515] -> w507
                tunnel: [w508 w516] -> w506
                tunnel: w504 -> [w509 w514]
                frame False {
                }
                frame True {
                  n177 = call "BaseSM.check state.vi"("i ref in"=w514, "error in (no error)"=w512) -> ("i ref out"=w513:refnum<vi>, "actualState"=w510:string, "error out"=w511:errorcluster)  [unwired: 12 in, 3 out]
                  n178 = case shown="Default" w510 {
                    tunnel: [w519 w534] -> w516
                    tunnel: [w520 w535] -> w515
                    tunnel: w513 -> [w524 w537]
                    tunnel: w511 -> [w523 w536]
                    frame Default {
                      n179 = call "PH_PowerUnit_BaseClass.get data to modify.vi"("i ref in"=w524, "error in (no error)"=w523) -> ("i ref out"=w521:refnum<vi>, "i attribute"=w517:T5, "timed out"=w518:bool, "error out"=w522:errorcluster)  [unwired: 14 in]
                      n180 = case shown="False" w518 {
                        tunnel: w522 -> [w531 w532]
                        tunnel: w521 -> [w530 w533]
                        tunnel: [w529 w533] -> w520
                        tunnel: [w528 w532] -> w519
                        tunnel: w517 -> [w527 _]
                        frame False {
                          n181 = Bundle By Name(cluster=w527, "PSDB data.Write 2 early"=TRUE) -> (w526:T5)
                          n182 = call "PH_PowerUnit_BaseClass.set modified data.vi"("i ref in"=w530, "i attribute"=w526, "error in (no error)"=w531) -> ("i ref out"=w529:refnum<vi>, "error out"=w528:errorcluster)  [unwired: 15 in]
                        }
                        frame True {
                        }
                      }
                    }
                    frame "Stand by", "Switch PU on", "Wait for Shot Cmd" {
                      n183 = call "PH_PPPA_PowerUnit.write PSDB.vi"("i ref in"=w537, "error IO"=w536) -> ("i ref out"=w538:refnum<vi>, "error out"=w539:errorcluster)  [unwired: 16 in]
                      n184 = call "PH_PSDBWriter.evt call write PSDB.vi"("i ref in"=w538, "error in (no error)"=w539) -> ("i ref out"=w535:refnum<vi>, "error out"=w534:errorcluster)  [unwired: 16 in]
                    }
                  }
                }
              }
            }
            frame Error {
            }
          }
          n185 = call "BaseProcess.set event status.vi"("i ref in"=w480, "EventStatus"=w489, "error in (no error)"=w479) -> ("i ref out"=w493:refnum<vi>, "error out"=w492:errorcluster)  [unwired: 14 in, 1 out]
          n186 = Unbundle By Name(w492) -> ("code"=w495:i32)
          n187 = case shown="No Error" w492 {
            selector: w492 -> [_ w544]
            tunnel: [_ w542] -> w494
            frame No Error {
            }
            frame Error {
              n188 = Unbundle By Name(w544) -> ("source"=w543:string)
              n189 = call-poly "CoreLib.data 2 byte array.vi"("string"=w543) -> ("byteArray out"=w542:T1)  [unwired: 18 in]
            }
          }
          n190 = Bundle By Name(cluster=w491, "Data"=w494, "Error #"=w495) -> (w490:T2)
        }
        frame "_SMStateSequencer" {
          n191 = call "CAEObj.unfold trend data.vi"("i ref in"=w548, "raw trend data"=w549) -> ("quality"=w550:i32, "no link"=w553:bool, "data"=w551:i8[], "typeDescriptor"=w552:string, "error out"=w554:errorcluster)  [unwired: 9 in, 4 out]
          n192 = case shown="No Error" w554 {
            tunnel: w547 -> [w570 w574]
            tunnel: [w564 w573] -> w546
            tunnel: [w562 w574] -> w545
            tunnel: w548 -> [w571 w573]
            tunnel: w553 -> [w569 _]
            tunnel: w552 -> [w567 _]
            tunnel: w551 -> [w568 _]
            tunnel: w550 -> [w566 _]
            frame No Error {
              n193 = call "PH_DIM.get String.vi"("no link"=w569, "typeDescriptor"=w567, "data"=w568, "quality"=w566) -> ("Output String"=w572:string)
              n194 = call "PH_PowerUnit_BaseClass.PC Seq SM.vi"("i ref in"=w571, "SM State"=w572, "no link"=w569, "error in"=w570) -> ("i ref out"=w565:refnum<vi>, "error out"=w563:errorcluster)  [unwired: 14 in]
              n195 = call "PH_PPPA_PowerUnit.Action Seq SM.vi"("VI in"=w565, "error in (no error)"=w563) -> ("VI out"=w564:refnum<vi>, "error out"=w562:errorcluster)  [unwired: 16 in]
            }
            frame Error {
            }
          }
          n196 = call "BaseProcess.set event status.vi"("i ref in"=w546, "EventStatus"=w555, "error in (no error)"=w545) -> ("i ref out"=w559:refnum<vi>, "error out"=w558:errorcluster)  [unwired: 14 in, 1 out]
          n197 = Unbundle By Name(w558) -> ("code"=w561:i32)
          n198 = case shown="No Error" w558 {
            selector: w558 -> [_ w577]
            tunnel: [_ w575] -> w560
            frame No Error {
            }
            frame Error {
              n199 = Unbundle By Name(w577) -> ("source"=w576:string)
              n200 = call-poly "CoreLib.data 2 byte array.vi"("string"=w576) -> ("byteArray out"=w575:T1)  [unwired: 18 in]
            }
          }
          n201 = Bundle By Name(cluster=w557, "Data"=w560, "Error #"=w561) -> (w556:T2)
        }
        frame Default {
          n202 = call "PH_PowerUnit_BaseClass.ProcCases.vi"("i ref in"=w585, "selector"=w580, "Data"=w579, "call cluster"=w578, "error in (no error)"=w583) -> ("i ref out"=w587:refnum<vi>, "answer cluster"=w581:T2, "error out"=w586:errorcluster)  [unwired: 12 in]
          n203 = call "PH_PPPA_PowerUnit.Calc State PU.vi"("i ref in"=w587, "error in (no error)"=w586) -> ("i ref out"=w584:refnum<vi>, "error out"=w582:errorcluster)  [unwired: 16 in]
        }
      }
    }
    frame Error {
    }
  }
  "answer cluster" <- w7
  "i ref out" <- w4
  "error out" <- w3
